vi "Launch MFC.vi"(8 "error in":errorcluster, 11 "TEC Controller in":refnum<class "TEC Controller.lvclass">) -> (0 "error out":errorcluster, 2 "ID":string, 3 "TEC Controller out":refnum<class "TEC Controller.lvclass">)   [LabVIEW 2014, in "Humidifier Test Lib.lvlib" / "TEC Controller.lvclass"]
uses:
  TEC Controller.lvclass
  reusable/Session APIs/File Access/Config Data/Config Data.lvclass
  <userlib>/_Session Fwk/Session - Root.lvclass
  reusable/DAQ Device/Device/Device.lvclass
  reusable/Session APIs/Session Log/System Log.lvclass
  Devices/Alicat/Session Based/Alicat Device.lvclass
  Messages for Controller/Update Data MSG/Update Humidifier Controller MSG.lvclass
  <vilib>/Utility/config.llb/NI_LVConfig.lvlib
  <vilib>/Utility/config.llb/Read Key (Double).vi
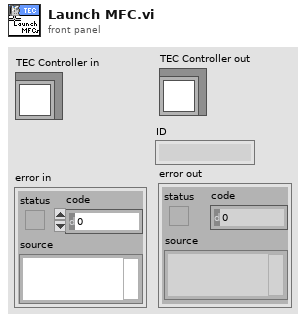
[diagram p1: front panel]
types:
  T1 = typedef "Session - Root.lvclass/Session Handle.ctl" = refnum<data-value>
  T2 = typedef "NI_LVConfig.lvlib/Config Data RefNum.ctl" = refnum<k1>
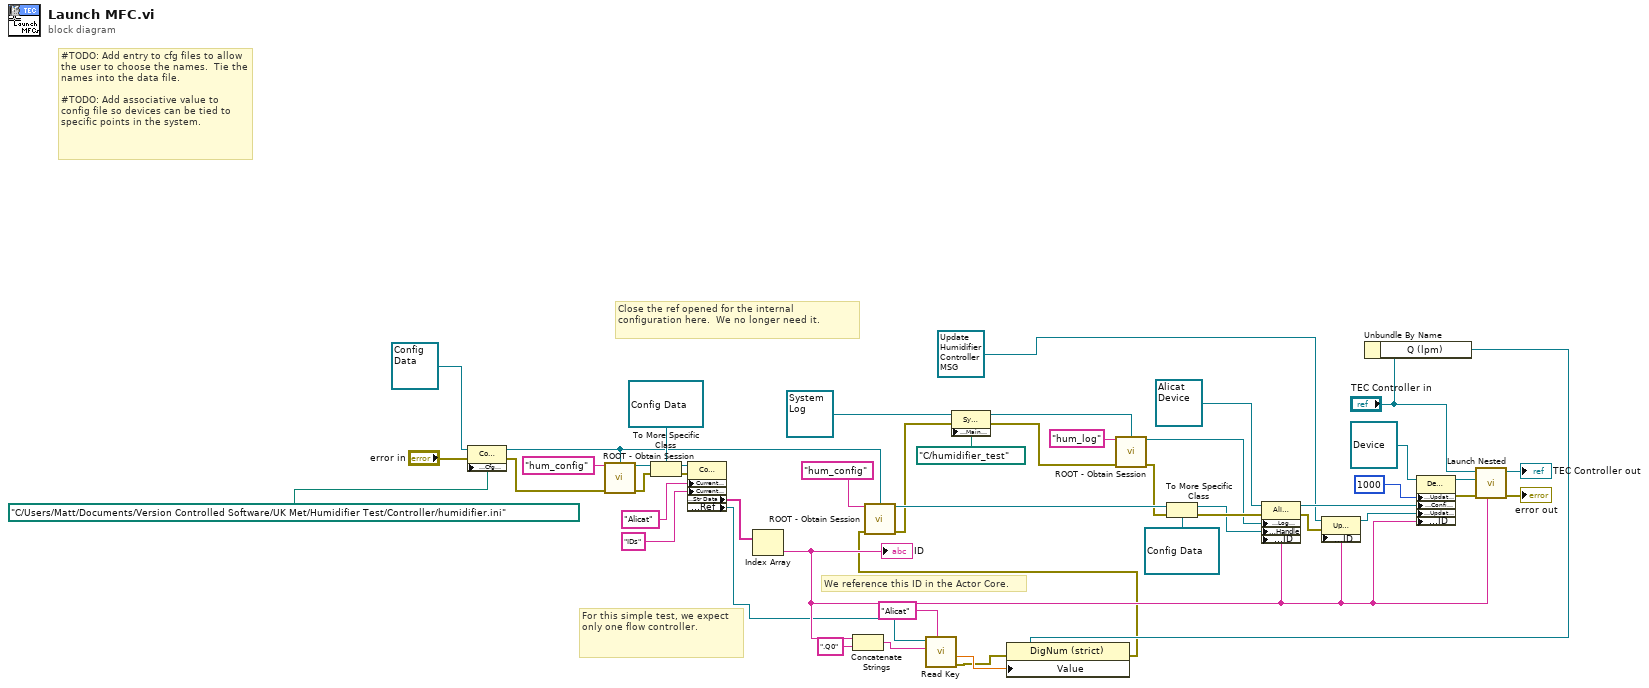
[diagram p0: block diagram]
diagram:
  # "We reference this ID in the Actor Core."
  # "Close the ref opened for the internal configuration here.  We no longer need it."
  # "For this simple test, we expect only one flow controller."
  # "#TODO: Add entry to cfg files to allow the user to choose the names.  Tie the names into the data file.\n\n#TODO: Add associative value to config file so devices can be tied to specific points in the system."
  n1 = property class="Config Data"(reference=refnum<class "Config Data.lvclass"> refnum ("Config Data"), error in="error in", "Accessors:Cfg Path"=path "C:/Users/Matt/Documents/Version Controlled Software/UK Met/Humidifier Test/Controller/humidifier.ini" ("Main Path")) -> (reference out=w40:refnum<class "Config Data.lvclass">, error out=w20:errorcluster)
  n2 = call <userlib>:"ROOT - Obtain Session.vi"("Session Name ()"="hum_config", "OBJ - Session"=w40, "error in (no error)"=w20) -> ("Session Handle"=w46:T1, "error out"=w37:errorcluster)  [unwired: 10 in, 1 out]
  n3 = To More Specific Class(target class=refnum<data-value> refnum ("Session Handle"), reference=w46, error in=w37) -> (specific class reference=w44:refnum<data-value>, error out=w19:errorcluster)
  n4 = property class="Config Data"(reference=w44, error in=w19, "Current Section"="Alicat", "Current Key"="IDs") -> ("Read Array Data:Str Data"=w41:string[], "Accessors:Ref"=w7:T2)  [unwired: 2 out]
  n5 = Index Array(array=w41) -> (element=w10:string)  [unwired: 1 in]
  "ID" <- w10
  n6 = Concatenate Strings(w10, ".Q0" ("string")) -> (w8:string)
  n7 = call-poly <vilib>:"Read Key.vi"("section"="Alicat", "key"=w8, "refnum"=w7) -> ("error out"=w2:errorcluster, "value"=w3:dbl)  [unwired: 5 in, 2 out]
  n8 = Unbundle By Name("TEC Controller in") -> ("Q (lpm)"=w4:refnum<vi>)
  n9 = property class="DigNum (strict)"(reference=w4, error in=w2, "Value"=w3) -> (error out=w1:errorcluster)  [unwired: 1 out]
  n10 = call <userlib>:"ROOT - Obtain Session.vi"("Session Name ()"="hum_config", "OBJ - Session"=w40, "error in (no error)"=w1) -> ("Session Handle"=w34:T1, "error out"=w17:errorcluster)  [unwired: 10 in, 1 out]
  n11 = property class="Sys Log"(reference=refnum<class "System Log.lvclass"> refnum ("Sys Log"), error in=w17, "Accessors:Main Path"=path "C:/humidifier_test" ("Main Path")) -> (reference out=w38:refnum<class "System Log.lvclass">, error out=w18:errorcluster)
  n12 = call <userlib>:"ROOT - Obtain Session.vi"("Session Name ()"="hum_log", "OBJ - Session"=w38, "error in (no error)"=w18) -> ("Session Handle"=w15:T1, "error out"=w16:errorcluster)  [unwired: 10 in, 1 out]
  n13 = To More Specific Class(target class=refnum<data-value> refnum ("Session Handle"), reference=w34, error in=w16) -> (specific class reference=w14:refnum<data-value>, error out=w32:errorcluster)
  n14 = property class="Alicat Device"(reference=refnum<class "Alicat Device.lvclass"> refnum ("Alicat Device in"), error in=w32, "Accessors:Log Session"=w15, "Accessors:Handle"=w14, "Accessors:ID"=w10) -> (reference out=w48:refnum<class "Alicat Device.lvclass">, error out=w13:errorcluster)
  n15 = property class="Update Humidifier Controller"(reference=refnum<class "Update Humidifier Controller MSG.lvclass"> refnum ("Humidifier Test Lib.lvlib:Update Humidifier Controller"), error in=w13, "Accessors:ID"=w10) -> (reference out=w12:refnum<class "Update Humidifier Controller MSG.lvclass">)  [unwired: 1 out]
  n16 = property class="Device"(reference=refnum<class "Device.lvclass"> refnum ("DAQ Device.lvlib:Device"), "Accessors:Update Period"=1000 ("Update Period"), "Accessors:Configurable Device"=w48, "Accessors:Update MSG"=w12, "Accessors:ID"=w10) -> (reference out=w29:refnum<class "Device.lvclass">, error out=w28:errorcluster)  [unwired: 1 in]
  n17 = call "Launch Nested.vi"("ID"=w10, "error in (no error)"=w28, "Nested Actor"=w29, "TEC Controller in"="TEC Controller in") -> ("error out"=→"error out":errorcluster, "TEC Controller out"=→"TEC Controller out":refnum<class "TEC Controller.lvclass">)  [unwired: 6 in]
